vi "encode DM.vi"(8 "error in (no error)":errorcluster, 10 "serial":string, 11 "RSeries_CAM in":refnum<class "RSeries_CAM.lvclass">) -> (0 "error out":errorcluster, 2 "DM":string, 3 "RSeries_CAM out":refnum<class "RSeries_CAM.lvclass">)   [LabVIEW 2024, in "RSeries_CAM.lvlib" / "RSeries_CAM.lvclass"]
uses:
  RSeries_CAM.lvclass
  RSeries_CAM.lvclass/RSeries_CAM.ctl
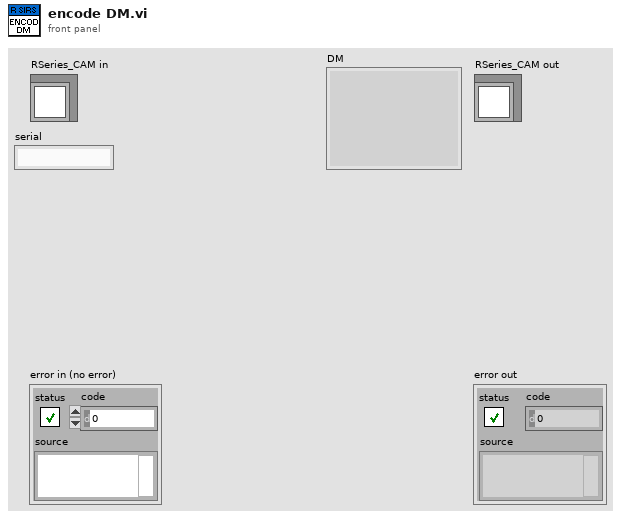
[diagram p1: front panel]
types:
  T1 = typedef "Open Batch Data.ctl" = cluster{"Batch Name":string, "Batch Number":string, "GTIN":string, "Expiry Date":string, "MFG Date":string}
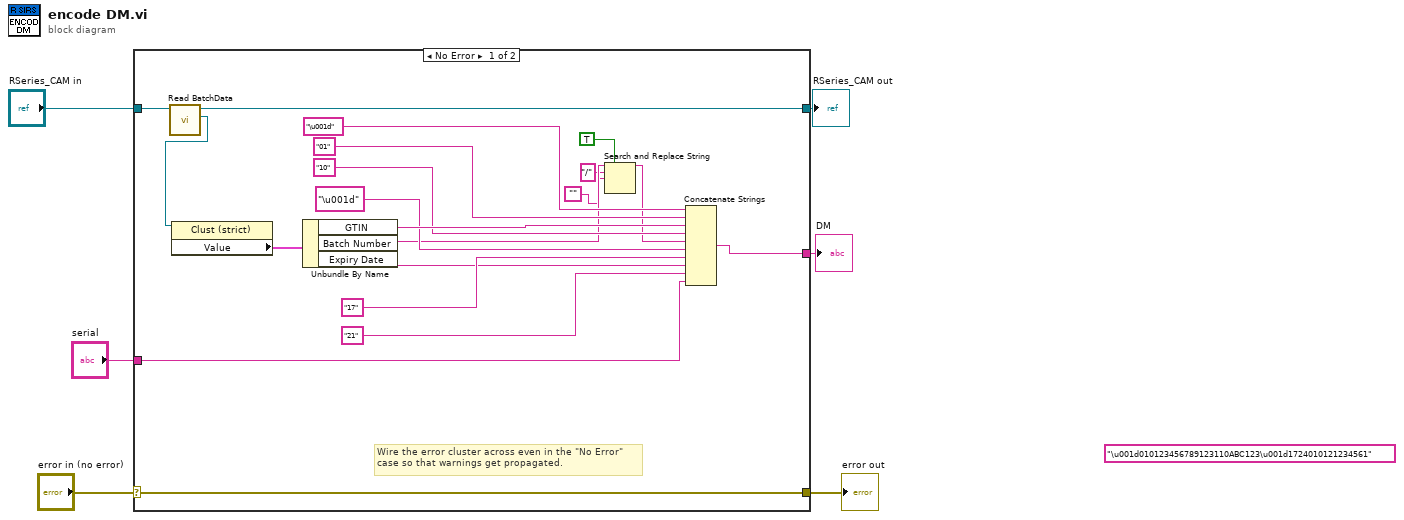
[diagram p0: block diagram]
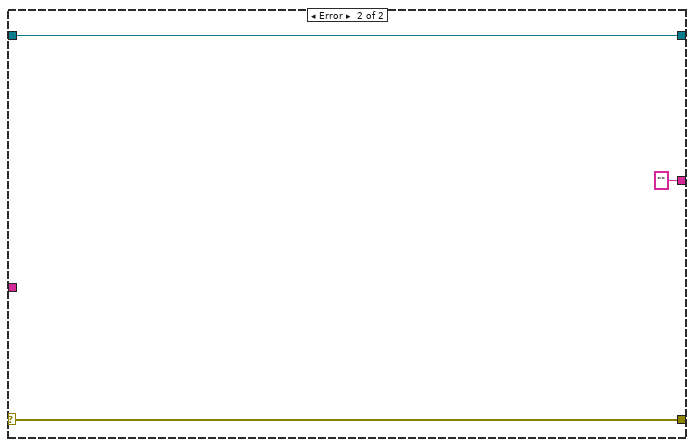
[diagram p2: hidden frame]
diagram:
  (unwired) "\u001d010123456789123110ABC123\u001d1724010121234561"
  n1 = case shown="No Error" "error in (no error)" {
    selector: "error in (no error)" -> [w26 w29]
    tunnel: [w26 w29] -> w5
    tunnel: "RSeries_CAM in" -> [w10 w28]
    tunnel: "serial" -> [w12 _]
    tunnel: [w11 ""] -> w2
    tunnel: [w9 w28] -> w1
    frame No Error {
      # "Wire the error cluster across even in the \"No Error\"\ncase so that warnings get propagated."
      n2 = call "Read BatchData.vi"("RSeries_CAM in"=w10) -> ("BatchData"=w8:refnum<vi>, "RSeries_CAM out"=w9:refnum<class "RSeries_CAM.lvclass">)  [unwired: 8 in, 1 out]
      n3 = property class="Clust (strict)"(reference=w8) -> ("Value"=w7:T1)  [unwired: 1 in, 2 out]
      n4 = Unbundle By Name(w7) -> ("GTIN"=w24:string, "Batch Number"=w16:string, "Expiry Date"=w20:string)
      n5 = Search and Replace String(replace all?=TRUE ("replace all? (F)"), input string=w16, search string="/", replace string="") -> (result string=w15:string)  [unwired: 4 in, 3 out]
      n6 = Concatenate Strings("\u001d" ("string"), "01" ("string"), w24, "10" ("string"), w15, "\u001d" ("string"), "17" ("string"), w20, "21" ("string"), w12) -> (w11:string)
    }
    frame Error {
    }
  }
  "error out" <- w5
  "RSeries_CAM out" <- w1
  "DM" <- w2
